vi "SSHPiComm.vi"(5 "password":string, 6 "Task":enum16{"init", "read", "write", "close"}(ring)=enum."close", 7 "Username":string, 9 "Text to write":string="\n\n", 11 "EV3 IP Address":string="192.168.1.36") -> (2 "text read":string="ReadSSH", 3 "Connected?":bool=TRUE)   [LabVIEW 2019]
panel:
  out "source":string="\n\n"
  out "error out":errorcluster
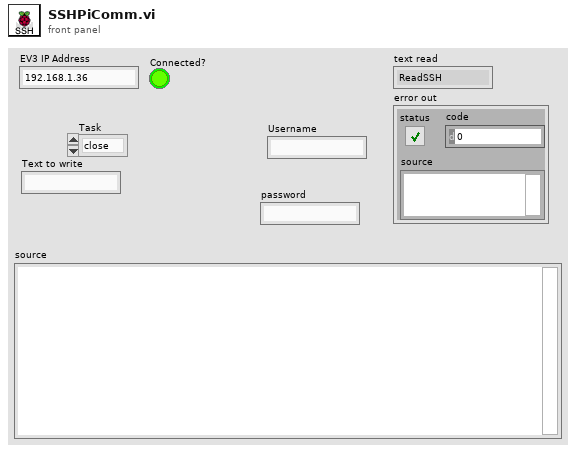
[diagram p1: front panel]
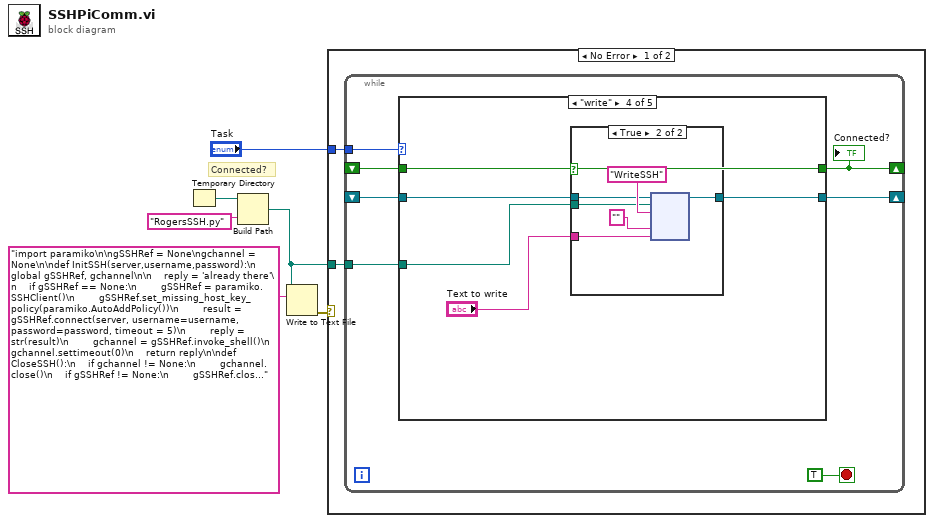
[diagram p0: block diagram]
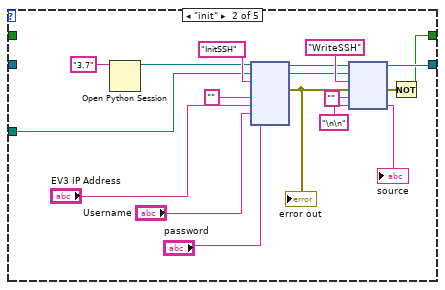
[diagram p3: hidden frame]
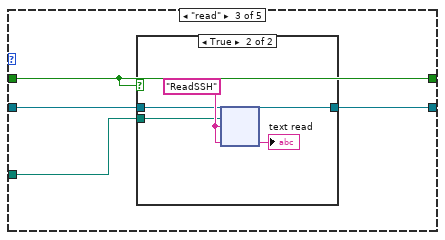
[diagram p4: hidden frame]
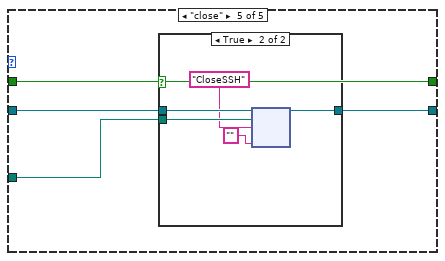
[diagram p7: hidden frame]
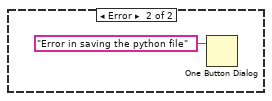
[diagram p9: hidden frame]
diagram:
  # "Connected?"
  n1 = Temporary Directory() -> (w4:path)
  n2 = Build Path(base path=w4, name or relative path="RogersSSH.py") -> (appended path=w3:path)
  n3 = Write to Text File(file (use dialog)=w3, text="import paramiko\n\ngSSHRef = None\ngchannel = None\n\ndef InitSSH(server,username,password):\n    global gSSHRef, gchannel\n\n    reply = 'already there'\n    if gSSHRef == None:\n        gSSHRef = paramiko.SSHClient()\n        gSSHRef.set_missing_host_key_policy(paramiko.AutoAddPolicy())\n        result = gSSHRef.connect(server, username=username, password=password, timeout = 5)\n        reply = str(result)\n        gchannel = gSSHRef.invoke_shell()\n        gchannel.settimeout(0)\n    return reply\n\ndef CloseSSH():\n    if gchannel != None:\n        gchannel.close()\n    if gSSHRef != None:\n        gSSHRef.close()\n    return('done')\n\ndef WriteSSH(string):\n    reply = 'no reference'\n    if gSSHRef != None:\n        reply = 'no file'\n        if gchannel != None:\n            size = gchannel.send(string.encode())\n            reply = str(size)\n    return reply\n\ndef ReadSSH():\n    reply = 'no reference'\n    if gSSHRef != None:\n        reply = 'no file'\n        if gchannel != None:\n            reply = ''\n            if gchannel.recv_ready():\n                reply = gchannel.recv(9999).decode()\n\n    return(reply)\n" ("name or relative path")) -> (error out=w1:errorcluster)  [unwired: 2 in, 2 out]
  n4 = case shown="No Error" w1 {
    tunnel: "Task" -> [w8 _]
    tunnel: w3 -> [w7 _]
    frame No Error {
      n5 = while {
        shift-right: [w15] -> _
        shift-left: _ -> [w13]
        tunnel: w8 -> [w14]
        tunnel: w7 -> [w12]
        shift-right: [w10] -> _
        shift-left: _ -> [w9]
        stop <- TRUE stop-if-true
        n6 = case shown="\"write\"" w14 {
          tunnel: [w17 w24 w37 w47 w59] -> w15
          tunnel: w13 -> [w17 _ w38 w48 w60]
          tunnel: w12 -> [_ w23 w36 w46 w58]
          tunnel: [w16 w19 w35 w45 w57] -> w10
          tunnel: w9 -> [w16 _ w35 w45 w57]
          frame Default {
          }
          frame "init" {
            n7 = Open Python Session(python version="3.7" ("Python version")) -> (session out=w25:refnum<k35>)  [unwired: 2 in, 1 out]
            n8 = node(w25, w23, "InitSSH" ("function name"), "" ("function name"), "EV3 IP Address", "Username", "password") -> (w26:refnum<k35>, w21:errorcluster)  [unwired: 5 in, 2 out]
            "error out" <- w21
            n9 = node(w26, w23, "WriteSSH" ("function name"), w21, "" ("function name"), "\n\n" ("function name")) -> (w24:refnum<k35>, w20:errorcluster, →"source":string)  [unwired: 1 in, 2 out]
            n10 = Not(x=w20) -> (.not. x?=w19:bool)
          }
          frame "read" {
            n11 = case shown="True" w35 {
              tunnel: w38 -> [w39 w43]
              tunnel: [w39 w42] -> w37
              tunnel: w36 -> [_ w41]
              frame False {
              }
              frame True {
                w44 = "ReadSSH" ("function name")
                n12 = node(w43, w41, w44, w44) -> (w42:refnum<k35>, →"text read":string)  [unwired: 1 in, 3 out]
              }
            }
          }
          frame "write" {
            n13 = case shown="True" w45 {
              tunnel: "Text to write" -> [_ w56]
              tunnel: w48 -> [w50 w53]
              tunnel: [w50 w52] -> w47
              tunnel: w46 -> [_ w51]
              frame False {
              }
              frame True {
                n14 = node(w53, w51, "WriteSSH" ("function name"), "" ("function name"), w56) -> (w52:refnum<k35>)  [unwired: 3 in, 3 out]
              }
            }
          }
          frame "close" {
            n15 = case shown="True" w57 {
              tunnel: w60 -> [w61 w65]
              tunnel: [w61 w64] -> w59
              tunnel: w58 -> [_ w63]
              frame False {
              }
              frame True {
                n16 = node(w65, w63, "CloseSSH" ("function name"), "" ("function name")) -> (w64:refnum<k35>)  [unwired: 2 in, 3 out]
              }
            }
          }
        }
        "Connected?" <- w10
      }
    }
    frame Error {
      n17 = One Button Dialog(message="Error in saving the python file") -> ()  [unwired: 1 in, 1 out]
    }
  }
